vi "StringifiedData.vi"(8 "error in (no error)":errorcluster, 11 "LVObjectMsg in":refnum<class "LVObjectMsg.lvclass">) -> (0 "error out":errorcluster, 2 "Stringified Data":string, 3 "LVObjectMsg out":refnum<class "LVObjectMsg.lvclass">)   [LabVIEW 2017, in "LapDog.Messaging.v3.NativeTypes.lvlib" / "LVObjectMsg.lvclass"]
doc: "This VI is used for the message probe. Child classes may override it and provide the message data in string format or a short string describing the data the message contains. This string will be displayed in the probe window."
uses:
  LVObjectMsg.lvclass
  LVObjectMsg.lvclass/LVObjectMsg.ctl
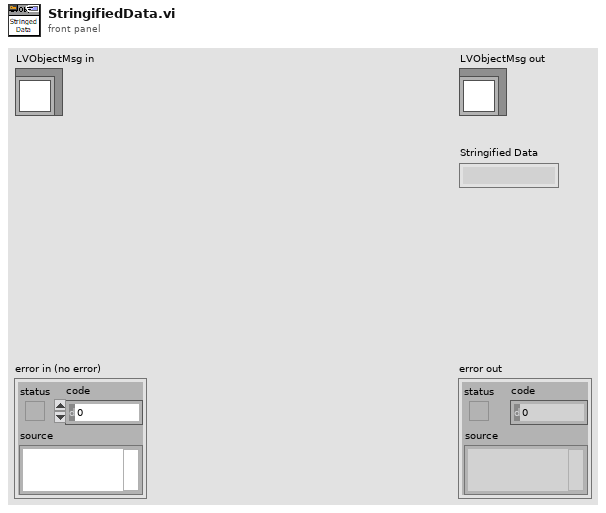
[diagram p1: front panel]
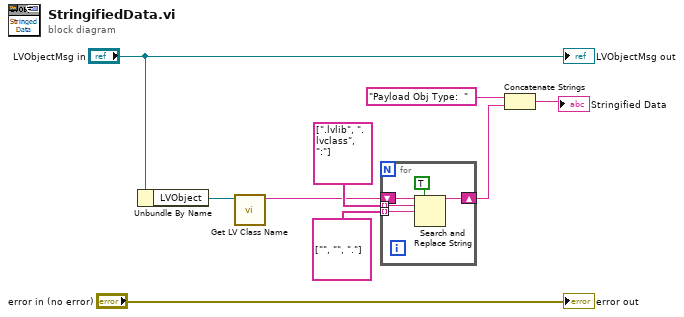
[diagram p0: block diagram]
diagram:
  n1 = Unbundle By Name("LVObjectMsg in") -> ("LVObject"=w7:refnum<class>)
  n2 = call <vilib>:"Get LV Class Name.vi"("object"=w7) -> ("class name"=w2:string)  [unwired: 9 in, 1 out]
  n3 = for {
    shift-right: [w12] -> w1
    shift-left: w2 -> [w14]
    tunnel: string[] [".lvlib", ".lvclass", ":"] -> [w11] mode=indexing
    tunnel: string[] ["", "", "."] -> [w10] mode=indexing
    n4 = Search and Replace String(replace all?=TRUE ("replace all? (F)"), input string=w14, search string=w11, replace string=w10) -> (result string=w12:string)  [unwired: 4 in, 3 out]
  }
  n5 = Concatenate Strings("Payload Obj Type:  " ("string"), w1) -> (→"Stringified Data":string)
  "error out" <- "error in (no error)"
  "LVObjectMsg out" <- "LVObjectMsg in"
